vi "Create HTML.vi"(7 "FP Reference":refnum<class "Web Front Panel.lvclass">, 8 "error in (no error)":errorcluster, 9 "Panel Origin":T1, 10 "VI Name":string, 11 "Object In":refnum<class "Object.lvclass">) -> (0 "error out":errorcluster, 1 "js code for controls":string, 2 "js variables":string, 3 "Object Out":refnum<class "Object.lvclass">, 4 "script dependencies":string[](array[string]), 5 "HTML":string, 6 "js code for indicators":string)   [LabVIEW 2015, in "Front Panel Publisher.lvlib" / "Object.lvclass"]
uses:
  Object.lvclass
  Web Front Panel_class/Web Front Panel.lvclass
  <vilib>/Utility/miscctls.llb/LVPointTypeDef.ctl
  Front Panel Publisher.lvlib
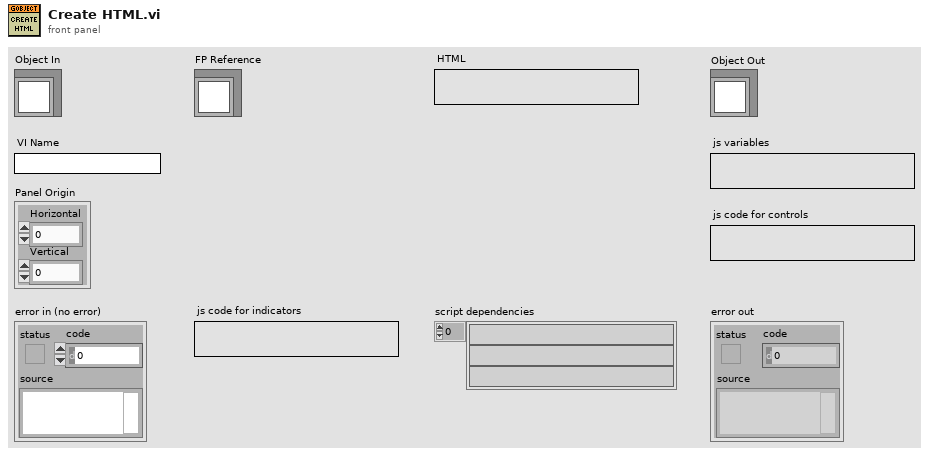
[diagram p1: front panel]
types:
  T1 = typedef "LVPointTypeDef.ctl" = cluster{"Horizontal":i16, "Vertical":i16}
  T2 = typedef "Front Panel Publisher.lvlib/Object.lvclass/Attributes.ctl" = cluster{"UID":i32, "Type":string, "Coordinates":T3, "Reference":refnum<vi>}
  T3 = typedef "Front Panel Publisher.lvlib/Object.lvclass/Coordinates.ctl" = cluster{"Left":i32, "Top":i32, "Height":u32, "Width":u32}
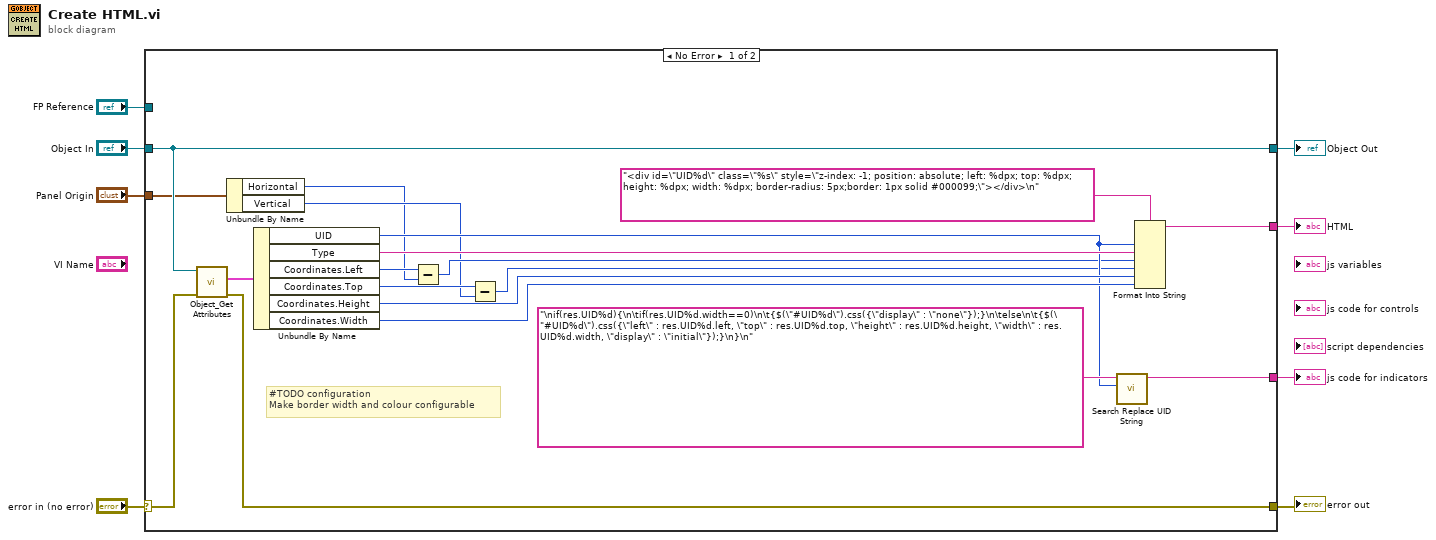
[diagram p0: block diagram]
diagram:
  n1 = case shown="No Error" "error in (no error)" {
    selector: "error in (no error)" -> [w27 w29]
    tunnel: [w26 w29] -> w7
    tunnel: [w17 w28] -> w5
    tunnel: "Object In" -> [w17 w28]
    tunnel: [w18 _] -> w4
    tunnel: "FP Reference" -> [_ _]
    tunnel: [w14 _] -> w2
    tunnel: "Panel Origin" -> [w11 _]
    frame No Error {
      # "#TODO configuration\nMake border width and colour configurable"
      n2 = call "Object_Get Attributes.vi"("error in (no error)"=w27, "Object In"=w17) -> ("error out"=w26:errorcluster, "Data"=w24:T2)  [unwired: 6 in, 2 out]
      n3 = Unbundle By Name(w11) -> ("Horizontal"=w9:i16, "Vertical"=w10:i16)
      n4 = Unbundle By Name(w24) -> ("UID"=w15:i32, "Type"=w23:string, "Coordinates.Left"=w22:i32, "Coordinates.Top"=w21:i32, "Coordinates.Height"=w20:u32, "Coordinates.Width"=w19:u32)
      n5 = Subtract(x=w22, y=w9) -> (x-y=w13:i32)
      n6 = Subtract(x=w21, y=w10) -> (x-y=w12:i32)
      n7 = call "Search Replace UID String.vi"("UID"=w15, "Input String"="\nif(res.UID%d){\n\tif(res.UID%d.width==0)\n\t{$(\"#UID%d\").css({\"display\" : \"none\"});}\n\telse\n\t{$(\"#UID%d\").css({\"left\" : res.UID%d.left, \"top\" : res.UID%d.top, \"height\" : res.UID%d.height, \"width\" : res.UID%d.width, \"display\" : \"initial\"});}\n}\n") -> ("Output String"=w14:string)  [unwired: 9 in]
      n8 = Format Into String(format string="<div id=\"UID%d\" class=\"%s\" style=\"z-index: -1; position: absolute; left: %dpx; top: %dpx; height: %dpx; width: %dpx; border-radius: 5px;border: 1px solid #000099;\"></div>\n", w15, w23, w13, w12, w20, w19) -> (resulting string=w18:string)  [unwired: 2 in, 1 out]
    }
    frame Error {
    }
  }
  "error out" <- w7
  "Object Out" <- w5
  "HTML" <- w4
  "js code for indicators" <- w2
